vi "Do.vi"(8 "error in (no error)":errorcluster, 10 "Actor in":refnum<class "Actor.lvclass">, 11 "Write Actor Filter Msg":refnum<class "Write Actor Filter Msg.lvclass">) -> (0 "error out":errorcluster, 2 "Actor out":refnum<class "Actor.lvclass">)   [LabVIEW 2016, in "CS++ObjectManager.lvlib" / "Write Actor Filter Msg.lvclass"]
doc: "This VI delivers the message to the actor by calling the appropriate method(s) on the actor."
uses:
  Write Actor Filter Msg.lvclass
  <vilib>/ActorFramework/Actor/Actor.lvclass
  CS++ObjectManager/CS++ObjectManager.lvclass
  C:/Program Files (x86)/National Instruments/LabVIEW 2016/vi.lib/ActorFramework/Actor/Actor.lvclass
  Write Actor Filter Msg.lvclass/Write Actor Filter Msg.ctl
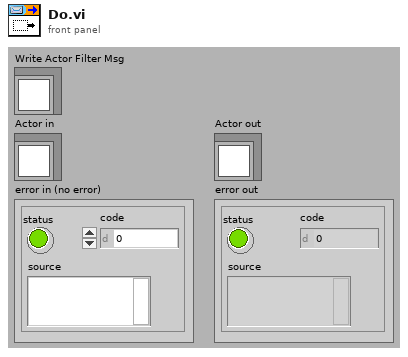
[diagram p1: front panel]
types:
  T1 = cluster{"PVMonitor":bool, "PVProxy":bool, "GUI":bool, "Other":bool}
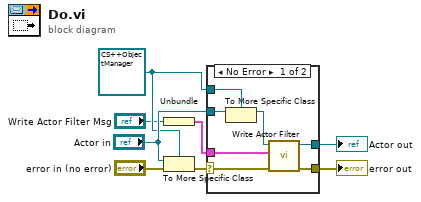
[diagram p0: block diagram]
diagram:
  w3 = refnum<class "CS++ObjectManager.lvclass"> refnum ("Actor in")
  n1 = Unbundle ("Main-Unbundle")("Write Actor Filter Msg") -> (w1:T1)
  n2 = To More Specific Class(target class=w3, reference="Actor in", error in="error in (no error)") -> (error out=w7:errorcluster)  [unwired: 1 out]
  n3 = case shown="No Error" w7 {
    selector: w7 -> [w13 w17]
    tunnel: [w15 w17] -> w6
    tunnel: [w14 w16] -> w5
    tunnel: "Actor in" -> [w12 w16]
    tunnel: w3 -> [w11 _]
    tunnel: w1 -> [w9 _]
    frame No Error {
      n4 = To More Specific Class(target class=w11, reference=w12) -> (specific class reference=w10:refnum<class "CS++ObjectManager.lvclass">)  [unwired: 1 in, 1 out]
      n5 = call-dynamic "Write Actor Filter.vi"("error in (no error)"=w13, "Actor Filter"=w9, "CS++ObjectManager in"=w10) -> ("error out"=w15:errorcluster, "CS++ObjectManager out"=w14:refnum<class "CS++ObjectManager.lvclass">)  [unwired: 7 in]
    }
    frame Error {
    }
  }
  "error out" <- w6
  "Actor out" <- w5
